vi "test Passes If Timestamps Are Equal.vi"(8 "error in (no error)":errorcluster, 11 "TestCase in":refnum<class "Timestamp Comparison Test Case.lvclass">) -> (0 "error out":errorcluster, 3 "TestCase out":refnum<class "Timestamp Comparison Test Case.lvclass">)   [LabVIEW 2015, in "Timestamp Comparison Test Case.lvclass"]
uses:
  Timestamp Comparison Test Case.lvclass
  <vilib>/addons/_JKI Toolkits/VI Tester/TestCase.llb/TestCase.lvclass
  VITAC.lvlib
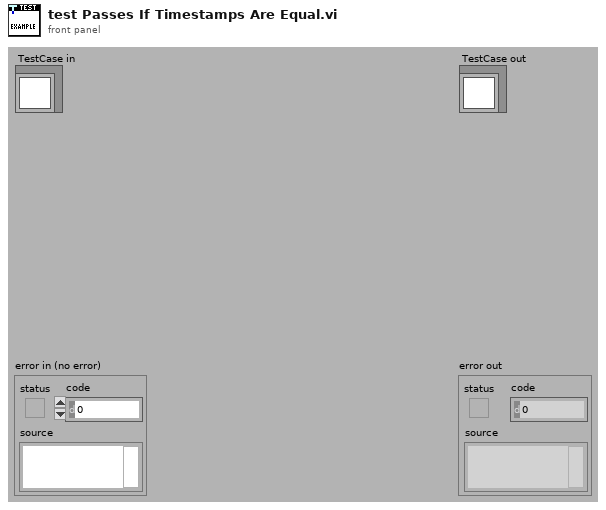
[diagram p1: front panel]
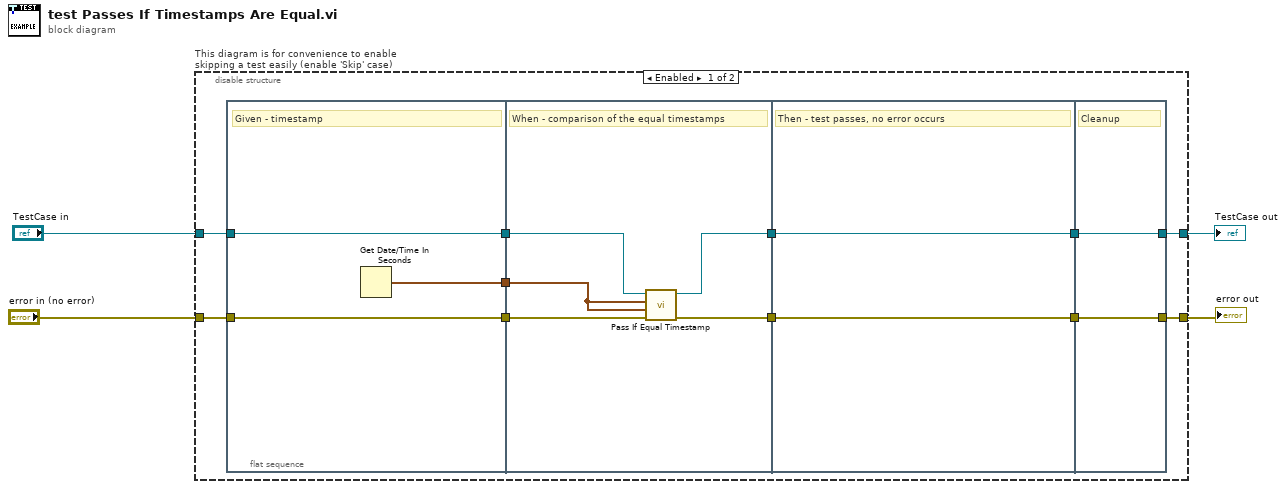
[diagram p0: block diagram]
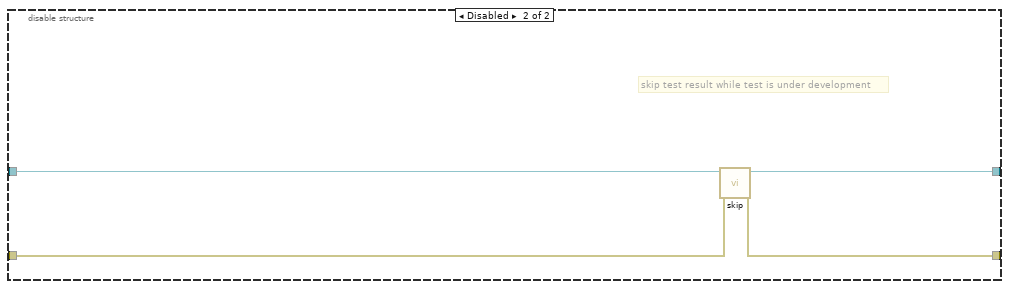
[diagram p2: hidden frame]
diagram:
  n1 = disable-structure "This diagram is for convenience to enable skipping a test easily (enable 'Skip' case)" shown="Enabled" {
    disable-tunnel: "TestCase in" -> [w7 w31]
    disable-tunnel: [w9 w29] -> w1
    disable-tunnel: [w8 w30] -> w3
    disable-tunnel: "error in (no error)" -> [w6 w28]
    frame Enabled {
      n2 = flat-sequence {
        tunnel: w6 -> [w17]
        tunnel: w7 -> [w18]
        tunnel: [w18] -> w15
        tunnel: [w17] -> w14
        tunnel: [w16] -> w5
        tunnel: [w20] -> w13
        tunnel: [w22] -> w12
        tunnel: w15 -> [w21]
        tunnel: w14 -> [w23]
        tunnel: w5 -> [w19]
        tunnel: [w25] -> w11
        tunnel: w13 -> [w25]
        tunnel: w12 -> [w24]
        tunnel: [w24] -> w10
        tunnel: [w26] -> w8
        tunnel: [w27] -> w9
        tunnel: w11 -> [w27]
        tunnel: w10 -> [w26]
        frame #0 {
          # "Given - timestamp"
          n3 = Get Date/Time In Seconds() -> (seconds since 1Jan1904=w16:timestamp)
        }
        frame #1 {
          # "When - comparison of the equal timestamps"
          n4 = call "Pass If Equal Timestamp.vi"("error in (no error)"=w23, "actual timestamp"=w19, "expected timestamp"=w19, "TestCase in"=w21) -> ("error out"=w22:errorcluster, "TestCase out"=w20:refnum<class "Timestamp Comparison Test Case.lvclass">)  [unwired: 6 in]
        }
        frame #2 {
          # "Then - test passes, no error occurs"
        }
        frame #3 {
          # "Cleanup"
        }
      }
    }
    frame Disabled {
      # "skip test result while test is under development"
      n5 = call <vilib>:"skip.vi"("error in (no error)"=w28, "TestCase in"=w31) -> ("error out"=w30:errorcluster, "TestCase out"=w29:refnum<class "Timestamp Comparison Test Case.lvclass">)  [unwired: 8 in]
    }
  }
  "error out" <- w3
  "TestCase out" <- w1
